vi "Keithley DC power manual control.vi"(8 "error in (no error)":errorcluster, 10 "DC power manual control":T1={"Channel Select"=enum."Channel 1", "Voltage (V)"=0.0, "Function(0:Voltage)"=0, "Current (mA)"=0.0, "Enable Output"=TRUE} {"Current (mA)" format="%.2f"; "Function(0:Voltage)" items=["Voltage", "Current"]; "Voltage (V)" format="%.2f"}, 11 "DC power COM":refnum<visa-resource-name>) -> (0 "error out":errorcluster, 3 "DC power COM":refnum<visa-resource-name>)   [LabVIEW 2017]
uses:
  <instrlib>/Keithley KE22xx Series/Keithley KE22xx Series.lvlib
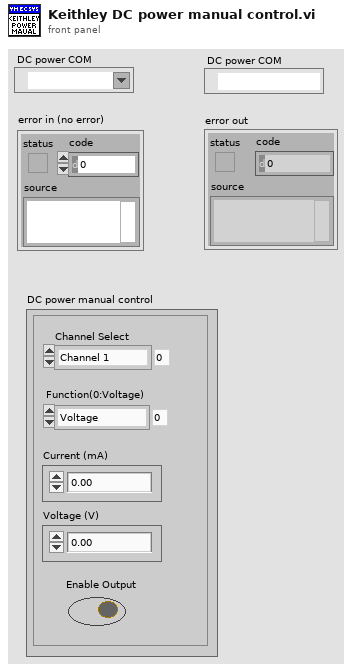
[diagram p1: front panel]
types:
  T1 = cluster{"Channel Select":enum16{"Channel 1", "Channel 2", "Channel 3"}, "Voltage (V)":dbl, "Function(0:Voltage)":u16, "Current (mA)":dbl, "Enable Output":bool}
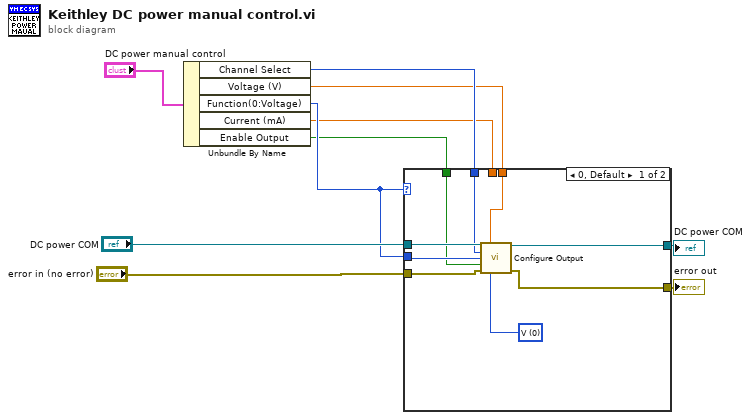
[diagram p0: block diagram]
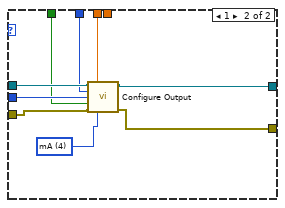
[diagram p2: hidden frame]
diagram:
  n1 = Unbundle By Name("DC power manual control") -> ("Channel Select"=w5:enum16{"Channel 1", "Channel 2", "Channel 3"}, "Voltage (V)"=w1:dbl, "Function(0:Voltage)"=w4:u16, "Current (mA)"=w2:dbl, "Enable Output"=w3:bool)
  n2 = case shown="0, Default" w4 {
    tunnel: "DC power COM" -> [w19 w28]
    tunnel: [w15 w27] -> w9
    tunnel: [w16 w26] -> w8
    tunnel: "error in (no error)" -> [w17 w25]
    tunnel: w5 -> [w14 w23]
    tunnel: w4 -> [w13 w22]
    tunnel: w3 -> [w12 w21]
    tunnel: w2 -> [_ w20]
    tunnel: w1 -> [w11 _]
    frame 0, Default {
      w18 = u16 0 items=["V", "mV", "kV", "A", "mA"] ("Unit(V)")
      n3 = call <instrlib>:"Configure Output.vi"("VISA resource name"=w19, "Manual Range(0.00)"=w11, "Channel Select"=w14, "Function(0:Voltage)"=w13, "Enable Output (T: Enable)"=w12, "error in (no error)"=w17, "Unit(V)"=w18) -> ("VISA resource name out"=w15:refnum<visa-resource-name>, "error out"=w16:errorcluster)  [unwired: 7 in]
    }
    frame 1 {
      w24 = u16 4 items=["V", "mV", "kV", "A", "mA"] ("Unit(V)")
      n4 = call <instrlib>:"Configure Output.vi"("VISA resource name"=w28, "Manual Range(0.00)"=w20, "Channel Select"=w23, "Function(0:Voltage)"=w22, "Enable Output (T: Enable)"=w21, "error in (no error)"=w25, "Unit(V)"=w24) -> ("VISA resource name out"=w27:refnum<visa-resource-name>, "error out"=w26:errorcluster)  [unwired: 7 in]
    }
  }
  "DC power COM" <- w9
  "error out" <- w8
